vi "Query with 1D Integer Result.vi"(8 "error in (no error)":errorcluster, 10 "Query string":string, 11 "sqlite3 in":refnum<class "sqlite3.lvclass">) -> (0 "error out":errorcluster, 2 "Result":i32[](array[numeric]), 3 "sqlite3 out":refnum<class "sqlite3.lvclass">)   [LabVIEW 2020, in "sqlite3.lvlib" / "sqlite3.lvclass"]
uses:
  sqlite3.lvclass
  sqlite3.lvclass/sqlite3.ctl
  541d2037-599a-4170-a209-c77a8b970395.vi
  sqlite/VIs/open v2.vi
  sqlite/VIs/close v2.vi
  sqlite/VIs/prepare v2.vi
  sqlite/VIs/step.vi
  sqlite/VIs/column count.vi
  db layer/compound/Resolve Result Type.vi
  541d2037-599a-4170-a209-c77a8b970395.vi/0d0a347e-c06c-4fe3-8bbd-a0e3cf8c8a16.vi
  541d2037-599a-4170-a209-c77a8b970395.vi/c436ca37-bab3-4c10-9ba2-710cece85bd5.vi
  sqlite/VIs/finalize.vi
  sqlite/subvi/Error Converter (ErrCode or Status).vi
  sqlite/VIs/column type.vi
  sqlite/VIs/column int.vi
  541d2037-599a-4170-a209-c77a8b970395.vi/0d0a347e-c06c-4fe3-8bbd-a0e3cf8c8a16.vi/e2175d81-4f24-490a-8437-0be1725fd2b2.vi
  sqlite/VIs/errstr.vi
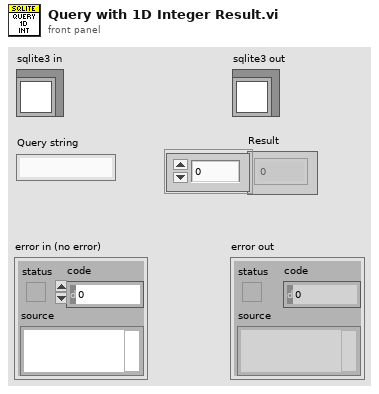
[diagram p1: front panel]
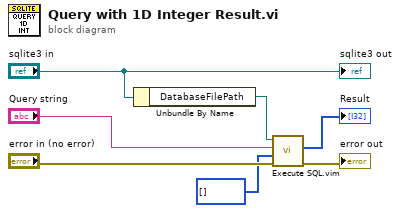
[diagram p0: block diagram]
diagram:
  n1 = Unbundle By Name("sqlite3 in") -> ("DatabaseFilePath"=w7:path)
  n2 = call "Execute SQL.vim"("error in (no error)"="error in (no error)", "desired return type(none)"=i32[] [] ("Result 2"), "sql (string)"="Query string", "database in"=w7) -> ("error out"=→"error out":errorcluster, "Query Result"=→"Result":i32[])  [unwired: 6 in]
  "sqlite3 out" <- "sqlite3 in"
